vi "axis equal in labview.vi"(8 "y min":dbl, 9 "y max":dbl, 10 "x min":dbl, 11 "x max":dbl) -> (0 "yscale min":dbl, 1 "yscale max":dbl, 2 "xscale min":dbl, 3 "xscale max":dbl)   [LabVIEW 2015]
uses:
  <vilib>/Analysis/baseanly.llb/Mean (DBL).vi
  <vilib>/Analysis/NI_AALBase.lvlib
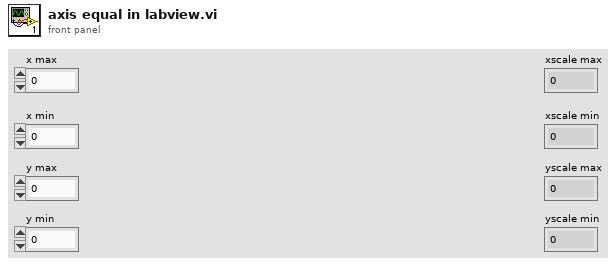
[diagram p1: front panel]
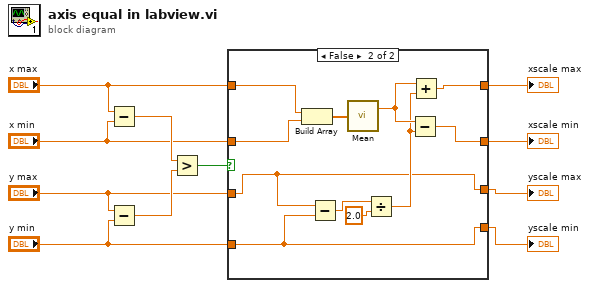
[diagram p0: block diagram]
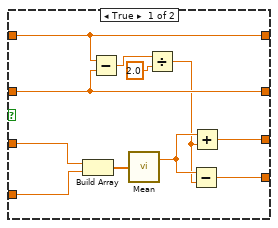
[diagram p2: hidden frame]
diagram:
  n1 = Subtract(x="x max", y="x min") -> (x-y=w11:dbl)
  n2 = Subtract(x="y max", y="y min") -> (x-y=w10:dbl)
  n3 = Greater?(x=w11, y=w10) -> (0:w9:bool)
  n4 = case shown="False" w9 {
    tunnel: [w22 w24] -> w4
    tunnel: "x max" -> [w22 w26]
    tunnel: [w21 w23] -> w3
    tunnel: "x min" -> [w21 w25]
    tunnel: "y max" -> [w17 w28]
    tunnel: "y min" -> [w16 w27]
    tunnel: [w13 w28] -> w2
    tunnel: [w12 w27] -> w1
    frame True {
      n5 = Build Array(w17, w16) -> (w18:dbl[])
      n6 = Subtract(x=w22, y=w21) -> (x-y=w20:dbl)
      n7 = call-poly <vilib>:"Mean.vi"("X"=w18) -> ("mean"=w15:dbl)  [unwired: 1 out]
      n8 = Divide(x=w20, y=2.0) -> (x/y=w14:dbl)
      n9 = Subtract(x=w15, y=w14) -> (x-y=w12:dbl)
      n10 = Add(x=w15, y=w14) -> (x+y=w13:dbl)
    }
    frame False {
      n11 = Build Array(w26, w25) -> (w31:dbl[])
      n12 = Subtract(x=w28, y=w27) -> (x-y=w33:dbl)
      n13 = call-poly <vilib>:"Mean.vi"("X"=w31) -> ("mean"=w30:dbl)  [unwired: 1 out]
      n14 = Divide(x=w33, y=2.0) -> (x/y=w29:dbl)
      n15 = Subtract(x=w30, y=w29) -> (x-y=w23:dbl)
      n16 = Add(x=w30, y=w29) -> (x+y=w24:dbl)
    }
  }
  "xscale max" <- w4
  "xscale min" <- w3
  "yscale max" <- w2
  "yscale min" <- w1
